vi "userTable.vi"() -> ()   [LabVIEW 2020, in "userLibrary.lvlib"]
uses:
  userLibrary.lvlib
  <vilib>/Utility/miscctls.llb/LVRowAndColumnTypeDef.ctl
  <vilib>/measure/mamon.llb/Trigger Detection for 1 Channel.vi
  <vilib>/addons/database/Connection.llb/DB Tools Open Connec (String).vi
  <vilib>/addons/database/NI_Database_API.lvlib
  databaseLibrary.lvlib
  maintenanceLibrary.lvlib
  <vilib>/measure/NI_MAPro.lvlib
panel:
  in  "close":bool
  out "status 5":bool
  out "status 4":bool
  out "status 3":bool
  out "status 2":bool
  out "status 1":bool
  out "Log Max row":i32
  in  "OK":bool
  in  "Change Pass":bool
  out "data":string[][](array[string])
  in  "Delete":bool
  in  "Update":bool
  in  "New":bool
  out "User Table":string[][](table) caption="Thickness Table"
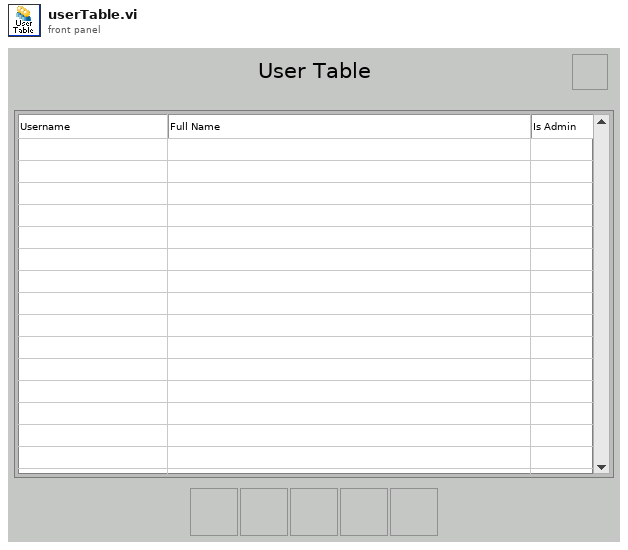
[diagram p1: front panel]
types:
  T1 = typedef "LVRowAndColumnTypeDef.ctl" = cluster{"Row":i32, "Column":i32}
  T2 = typedef "NI_Database_API.lvlib/Conn ObjectReference.ctl" = refnum<k1>
  T3 = cluster{"date/time string":string, "date/time string":string, "date/time string":string, string}
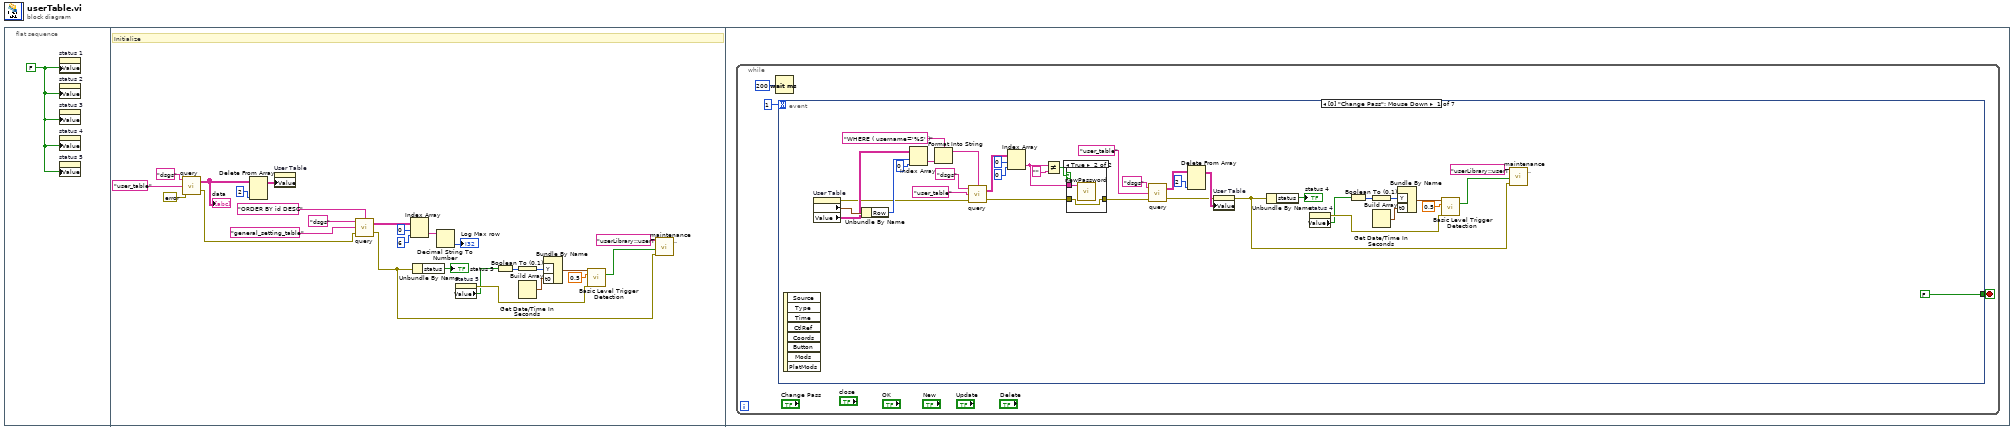
[diagram p0: block diagram]
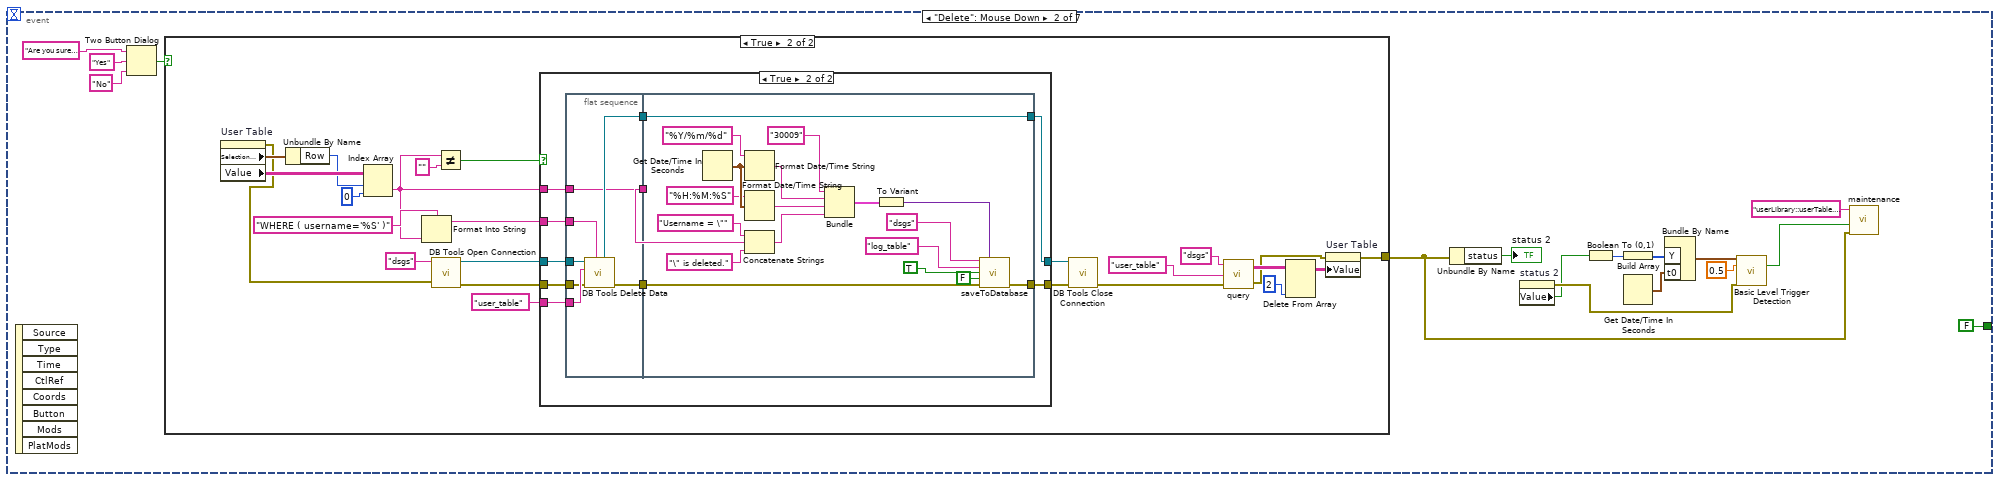
[diagram p3: hidden frame]
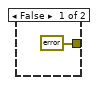
[diagram p4: hidden frame]
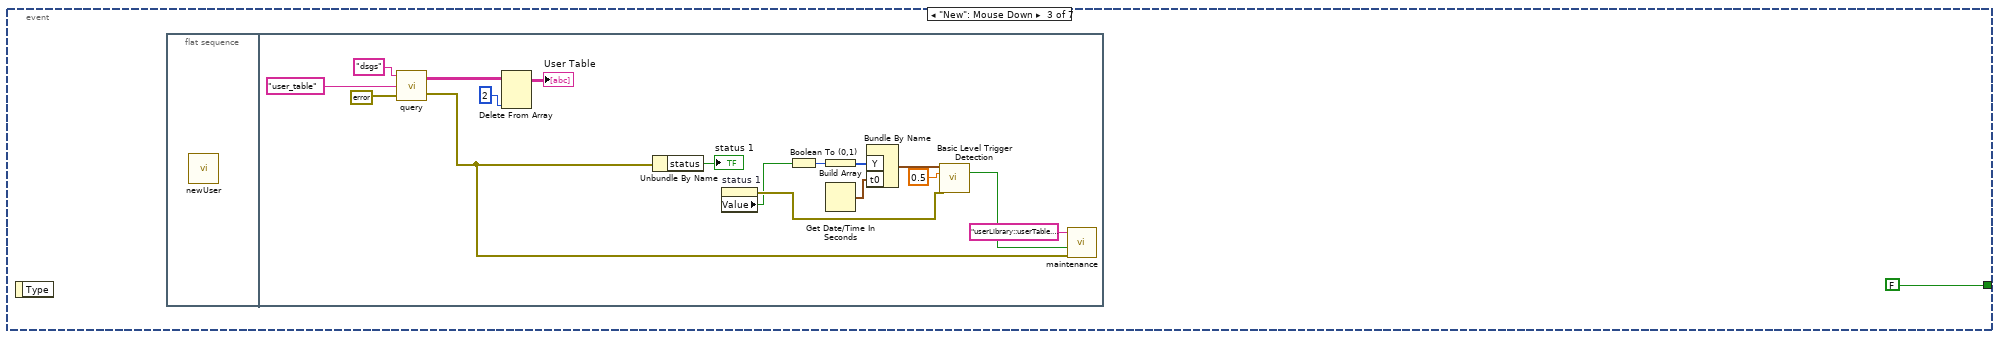
[diagram p6: hidden frame]
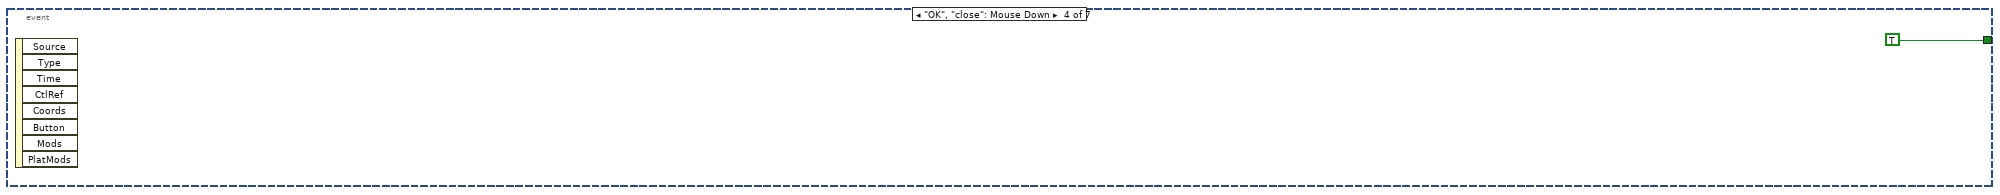
[diagram p7: hidden frame]
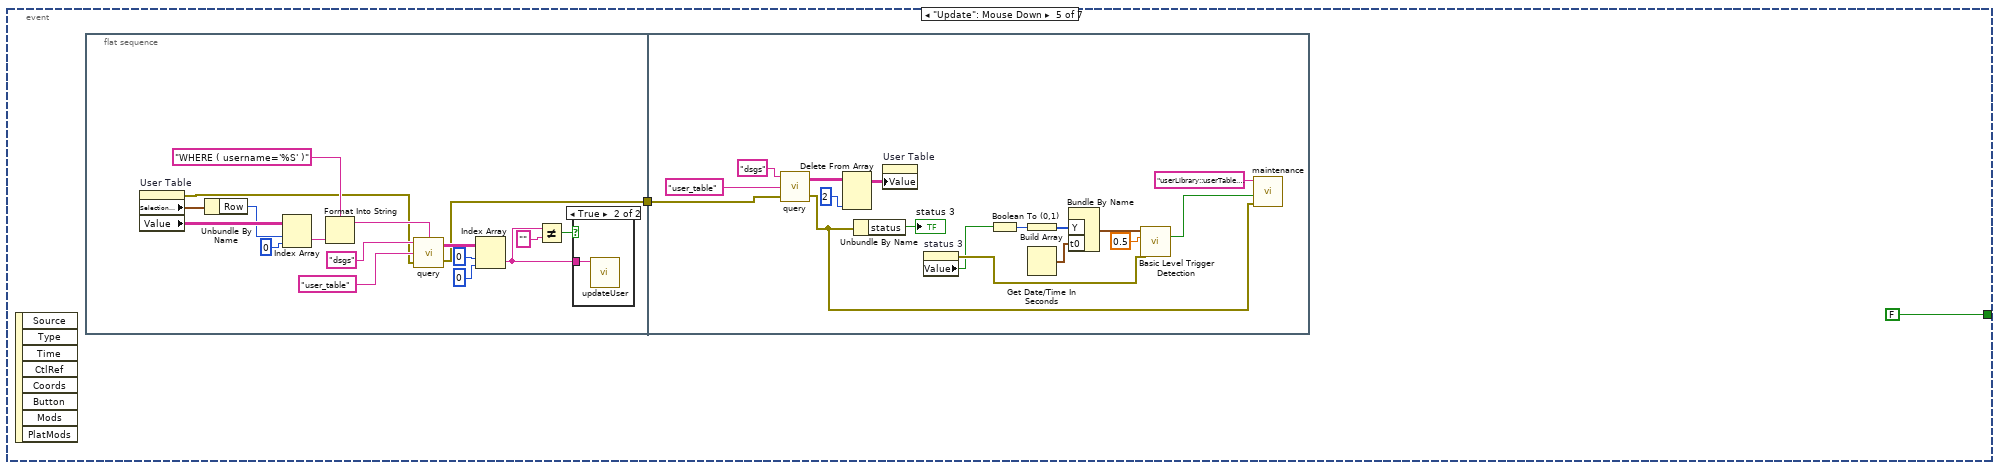
[diagram p8: hidden frame]
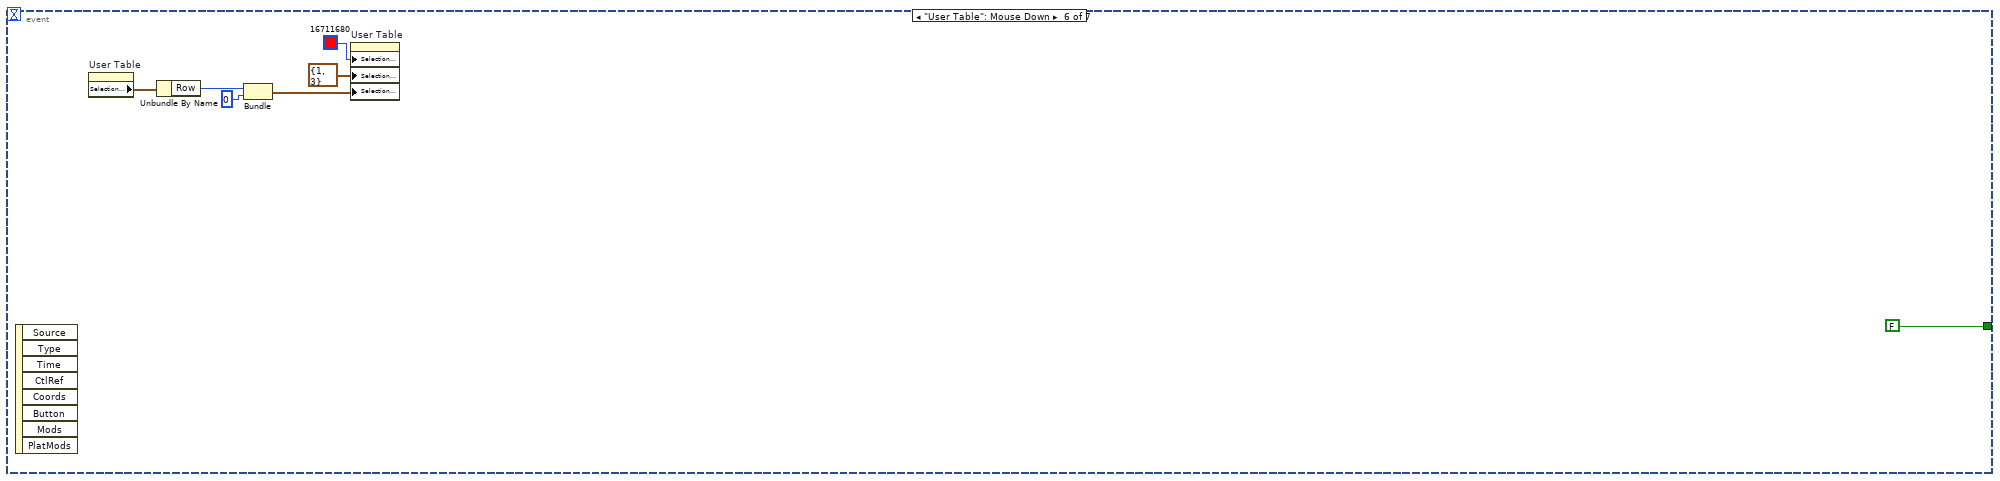
[diagram p10: hidden frame]
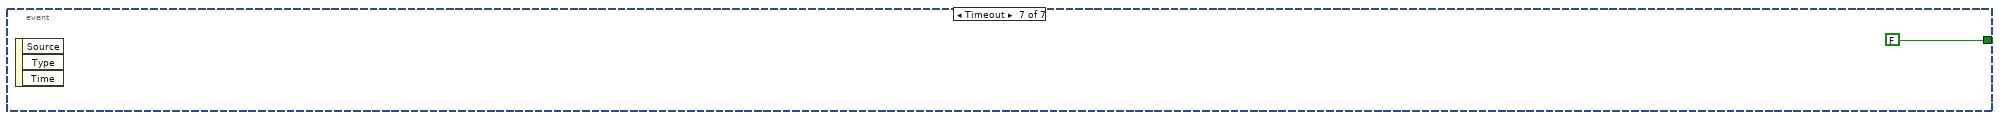
[diagram p11: hidden frame]
diagram:
  n1 = flat-sequence {
    frame #0 {
      w1 = FALSE ("status 1")
      n2 = property on="status 1" class="Bool (strict)"("Value"=w1) -> ()  [unwired: 2 in, 2 out]
      n3 = property on="status 2" class="Bool (strict)"("Value"=w1) -> ()  [unwired: 2 in, 2 out]
      n4 = property on="status 3" class="Bool (strict)"("Value"=w1) -> ()  [unwired: 2 in, 2 out]
      n5 = property on="status 4" class="Bool (strict)"("Value"=w1) -> ()  [unwired: 2 in, 2 out]
      n6 = property on="status 5" class="Bool (strict)"("Value"=w1) -> ()  [unwired: 2 in, 2 out]
    }
    frame #1 {
      # "Initialize"
      n7 = call "query.vi"("errorIn"=errorcluster {"status"=FALSE, "code"=0, "source"=""} ("Error in"), "Table Name"="user_table", "Connection Name"="dsgs") -> ("errorOut"=w14:errorcluster, "data"=w25:string[][])  [unwired: 1 in]
      "data" <- w25
      n8 = Delete From Array(array=w25, index (col)=2 ("disabled index (col)")) -> (array with subset deleted=w24:string[][])  [unwired: 2 in, 1 out]
      n9 = property on="User Table" class="Tbl (strict)"("Value"=w24) -> ()  [unwired: 2 in, 2 out]
      n10 = call "query.vi"("Condition"="ORDER BY id DESC", "errorIn"=w14, "Table Name"="general_setting_table", "Connection Name"="dsgs") -> ("errorOut"=w2:errorcluster, "data"=w22:string[][])
      n11 = Index Array(array=w22, index (row)=0, index (col)=6 ("disabled index (col)")) -> (element=w15:string)
      n12 = Unbundle By Name(w2) -> ("status"=→"status 5":bool)
      n13 = Decimal String To Number(string=w15) -> (number=→"Log Max row":i32)  [unwired: 2 in, 1 out]
      n14 = property on="status 5" class="Bool (strict)"() -> (error out=w10:errorcluster, "Value"=w9:bool)  [unwired: 2 in, 1 out]
      n15 = Boolean To (0,1)(Boolean=w9) -> (0, 1=w5:i16)
      n16 = Build Array(w5) -> (w7:i16[])
      n17 = Get Date/Time In Seconds() -> (seconds since 1Jan1904=w6:timestamp)
      n18 = Bundle By Name("Y"=w7, "t0"=w6) -> (w8:waveform(i16))  [unwired: 1 in]
      n19 = call-poly <vilib>:"Basic Level Trigger Detection.vi"("signal in"=w8, "level"=0.5, "error in (no error)"=w10) -> ("trigger detected?"=w11:bool)  [unwired: 10 in, 2 out]
      n20 = call "maintenance.vi"("errorIn"=w2, "status"=w11, "errorLocation"="userLibrary::userTable.vi::Initialize") -> ()  [unwired: 8 in, 1 out]
    }
    frame #2 {
      n21 = while {
        stop <- w28 stop-if-true
        n22 = Wait (ms)(milliseconds to wait=u32 200) -> ()  [unwired: 1 out]
        n23 = event shown="[0] \"Change Pass\": Mouse Down" {
          selector: _ -> [_ _ _ _ _ _ _]
          dyn-events: _ -> [_ _ _ _ _ _ _]
          timeout: 1 -> [_ _ _ _ _ _ _]
          tunnel: [FALSE FALSE FALSE TRUE FALSE FALSE FALSE] -> w28
          event "Change Pass": Mouse Down {
            n24 = event-data() -> ()  [unwired: 1 in, 8 out]
            n25 = property on="User Table" class="Tbl (strict)"() -> (error out=w43:errorcluster, "Selection Start"=w65:T1, "Value"=w64:string[][])  [unwired: 2 in, 1 out]
            n26 = Unbundle By Name(w65) -> ("Row"=w63:i32)
            n27 = Index Array(array=w64, index (row)=w63, index (col)=0 ("disabled index (col)")) -> (element=w66:string)
            n28 = Format Into String(format string="WHERE ( username='%S' )" ("condition"), w66) -> (resulting string=w60:string)  [unwired: 2 in, 1 out]
            n29 = call "query.vi"("Condition"=w60, "errorIn"=w43, "Table Name"="user_table", "Connection Name"="dsgs") -> ("errorOut"=w61:errorcluster, "data"=w59:string[][])
            n30 = Index Array(array=w59, index (row)=0, index (col)=0 ("disabled index (col)")) -> (element=w58:string)
            n31 = Not Equal?(x=w58, y="") -> (x != y?=w57:bool)
            n32 = case shown="True" w57 {
              tunnel: [w67 w68] -> w62
              tunnel: w61 -> [w67 w68]
              tunnel: w58 -> [_ w69]
              frame False {
              }
              frame True {
                n33 = call "newPassword.vi"("Username"=w69) -> ()  [unwired: 11 in]
              }
            }
            n34 = call "query.vi"("errorIn"=w62, "Table Name"="user_table", "Connection Name"="dsgs") -> ("errorOut"=w42:errorcluster, "data"=w56:string[][])  [unwired: 1 in]
            n35 = Delete From Array(array=w56, index (col)=2 ("disabled index (col)")) -> (array with subset deleted=w55:string[][])  [unwired: 2 in, 1 out]
            n36 = property on="User Table" class="Tbl (strict)"(error in=w42, "Value"=w55) -> (error out=w31:errorcluster)  [unwired: 1 in, 1 out]
            n37 = Unbundle By Name(w31) -> ("status"=→"status 4":bool)
            n38 = property on="status 4" class="Bool (strict)"() -> (error out=w39:errorcluster, "Value"=w38:bool)  [unwired: 2 in, 1 out]
            n39 = Boolean To (0,1)(Boolean=w38) -> (0, 1=w34:i16)
            n40 = Build Array(w34) -> (w36:i16[])
            n41 = Get Date/Time In Seconds() -> (seconds since 1Jan1904=w35:timestamp)
            n42 = Bundle By Name("Y"=w36, "t0"=w35) -> (w37:waveform(i16))  [unwired: 1 in]
            n43 = call-poly <vilib>:"Basic Level Trigger Detection.vi"("signal in"=w37, "level"=0.5, "error in (no error)"=w39) -> ("trigger detected?"=w40:bool)  [unwired: 10 in, 2 out]
            n44 = call "maintenance.vi"("errorIn"=w31, "status"=w40, "errorLocation"="userLibrary::userTable.vi::Change Pass case") -> ()  [unwired: 8 in, 1 out]
          }
          event "Delete": Mouse Down {
            n45 = event-data() -> ()  [unwired: 1 in, 8 out]
            n46 = Two Button Dialog(message="Are you sure to delete this user?", 1:"No" ("F button name (\"Cancel\")"), 2:"Yes" ("T button name (\"OK\")")) -> (T button?=w85:bool)
            n47 = case shown="True" w85 {
              tunnel: [errorcluster {"status"=FALSE, "code"=0, "source"=""} ("error out") w87] -> w70
              frame False {
              }
              frame True {
                n48 = property on="User Table" class="Tbl (strict)"() -> (error out=w89:errorcluster, "Selection Start"=w110:T1, "Value"=w105:string[][])  [unwired: 2 in, 1 out]
                n49 = Unbundle By Name(w110) -> ("Row"=w104:i32)
                n50 = Index Array(array=w105, index (row)=w104, index (col)=0 ("disabled index (col)")) -> (element=w90:string)
                n51 = Format Into String(format string="WHERE ( username='%S' )" ("condition"), w90) -> (resulting string=w97:string)  [unwired: 2 in, 1 out]
                n52 = call-poly <vilib>:"DB Tools Open Connection.vi"("error in (no error)"=w89, "connection information"="dsgs") -> ("error out"=w106:errorcluster, "connection reference"=w108:T2)  [unwired: 6 in]
                n53 = Not Equal?(x=w90, y="") -> (x != y?=w95:bool)
                n54 = case shown="True" w95 {
                  tunnel: w108 -> [w112 w122]
                  tunnel: "user_table" ("table") -> [_ w121]
                  tunnel: w106 -> [w111 w120]
                  tunnel: [w112 w119] -> w102
                  tunnel: [w111 w118] -> w101
                  tunnel: w97 -> [_ w117]
                  tunnel: w90 -> [_ w114]
                  frame False {
                  }
                  frame True {
                    n55 = flat-sequence {
                      tunnel: w122 -> [w129]
                      tunnel: w121 -> [w128]
                      tunnel: w120 -> [w127]
                      tunnel: w117 -> [w124]
                      tunnel: [w126] -> w116
                      tunnel: [w125] -> w115
                      tunnel: w114 -> [w123]
                      tunnel: [w123] -> w113
                      tunnel: [w136] -> w118
                      tunnel: [w148] -> w119
                      tunnel: w116 -> [w148]
                      tunnel: w115 -> [w131]
                      tunnel: w113 -> [w135]
                      frame #0 {
                        n56 = call <vilib>:"DB Tools Delete Data.vi"("condition"=w124, "error in (no error)"=w127, "table"=w128, "connection reference"=w129) -> ("error out"=w125:errorcluster, "connection reference out"=w126:T2)  [unwired: 6 in]
                      }
                      frame #1 {
                        n57 = Get Date/Time In Seconds() -> (seconds since 1Jan1904=w146:timestamp)
                        n58 = Format Date/Time String(time format string (%c)="%Y/%m/%d", seconds (now)=w146) -> (date/time string=w145:string)  [unwired: 1 in]
                        n59 = Format Date/Time String(time format string (%c)="%H:%M:%S", seconds (now)=w146) -> (date/time string=w144:string)  [unwired: 1 in]
                        n60 = Concatenate Strings("Username = \"" ("string"), w135, "\" is deleted." ("string")) -> (w147:string)
                        n61 = Bundle("date/time string"="30009", "date/time string"=w145, "date/time string"=w144, w147) -> (w143:T3)  [unwired: 1 in]
                        n62 = To Variant(anything=w143) -> (Variant=w142:variant)
                        n63 = call "saveToDatabase.vi"("Connection"="dsgs" ("table"), "Data"=w142, "Table"="log_table" ("table"), "Auto Increment ID?"=TRUE, "Delete row?"=FALSE, "Error in"=w131) -> ("Error out"=w136:errorcluster)  [unwired: 9 in]
                      }
                    }
                  }
                }
                n64 = call <vilib>:"DB Tools Close Connection.vi"("error in (no error)"=w101, "connection reference"=w102) -> ("error out"=w98:errorcluster)  [unwired: 5 in]
                n65 = call "query.vi"("errorIn"=w98, "Table Name"="user_table", "Connection Name"="dsgs") -> ("errorOut"=w88:errorcluster, "data"=w92:string[][])  [unwired: 1 in]
                n66 = Delete From Array(array=w92, index (col)=2 ("disabled index (col)")) -> (array with subset deleted=w91:string[][])  [unwired: 2 in, 1 out]
                n67 = property on="User Table" class="Tbl (strict)"(error in=w88, "Value"=w91) -> (error out=w87:errorcluster)  [unwired: 1 in, 1 out]
              }
            }
            n68 = Unbundle By Name(w70) -> ("status"=→"status 2":bool)
            n69 = property on="status 2" class="Bool (strict)"() -> (error out=w78:errorcluster, "Value"=w77:bool)  [unwired: 2 in, 1 out]
            n70 = Boolean To (0,1)(Boolean=w77) -> (0, 1=w73:i16)
            n71 = Build Array(w73) -> (w75:i16[])
            n72 = Get Date/Time In Seconds() -> (seconds since 1Jan1904=w74:timestamp)
            n73 = Bundle By Name("Y"=w75, "t0"=w74) -> (w76:waveform(i16))  [unwired: 1 in]
            n74 = call-poly <vilib>:"Basic Level Trigger Detection.vi"("signal in"=w76, "level"=0.5, "error in (no error)"=w78) -> ("trigger detected?"=w79:bool)  [unwired: 10 in, 2 out]
            n75 = call "maintenance.vi"("errorIn"=w70, "status"=w79, "errorLocation"="userLibrary::userTable.vi::Delete case") -> ()  [unwired: 8 in, 1 out]
          }
          event "New": Mouse Down {
            n76 = event-data() -> ()  [unwired: 1 in, 1 out]
            n77 = flat-sequence {
              frame #0 {
                n78 = call "newUser.vi"() -> ()  [unwired: 12 in]
              }
              frame #1 {
                n79 = call "query.vi"("errorIn"=errorcluster {"status"=FALSE, "code"=0, "source"=""} ("Error in"), "Table Name"="user_table", "Connection Name"="dsgs") -> ("errorOut"=w150:errorcluster, "data"=w164:string[][])  [unwired: 1 in]
                n80 = Delete From Array(array=w164, index (col)=2 ("disabled index (col)")) -> (array with subset deleted=→"User Table":string[][])  [unwired: 2 in, 1 out]
                n81 = Unbundle By Name(w150) -> ("status"=→"status 1":bool)
                n82 = property on="status 1" class="Bool (strict)"() -> (error out=w158:errorcluster, "Value"=w157:bool)  [unwired: 2 in, 1 out]
                n83 = Boolean To (0,1)(Boolean=w157) -> (0, 1=w153:i16)
                n84 = Build Array(w153) -> (w155:i16[])
                n85 = Get Date/Time In Seconds() -> (seconds since 1Jan1904=w154:timestamp)
                n86 = Bundle By Name("Y"=w155, "t0"=w154) -> (w156:waveform(i16))  [unwired: 1 in]
                n87 = call-poly <vilib>:"Basic Level Trigger Detection.vi"("signal in"=w156, "level"=0.5, "error in (no error)"=w158) -> ("trigger detected?"=w159:bool)  [unwired: 10 in, 2 out]
                n88 = call "maintenance.vi"("errorIn"=w150, "status"=w159, "errorLocation"="userLibrary::userTable.vi::New case") -> ()  [unwired: 8 in, 1 out]
              }
            }
          }
          event "OK", "close": Mouse Down {
            n89 = event-data() -> ()  [unwired: 1 in, 8 out]
          }
          event "Update": Mouse Down {
            n90 = event-data() -> ()  [unwired: 1 in, 8 out]
            n91 = flat-sequence {
              tunnel: [w171] -> w168
              tunnel: w168 -> [w199]
              frame #0 {
                n92 = property on="User Table" class="Tbl (strict)"() -> (error out=w170:errorcluster, "Selection Start"=w186:T1, "Value"=w185:string[][])  [unwired: 2 in, 1 out]
                n93 = Unbundle By Name(w186) -> ("Row"=w184:i32)
                n94 = Index Array(array=w185, index (row)=w184, index (col)=0 ("disabled index (col)")) -> (element=w183:string)
                n95 = Format Into String(format string="WHERE ( username='%S' )" ("condition"), w183) -> (resulting string=w178:string)  [unwired: 2 in, 1 out]
                n96 = call "query.vi"("Condition"=w178, "errorIn"=w170, "Table Name"="user_table", "Connection Name"="dsgs") -> ("errorOut"=w171:errorcluster, "data"=w177:string[][])
                n97 = Index Array(array=w177, index (row)=0, index (col)=0 ("disabled index (col)")) -> (element=w174:string)
                n98 = Not Equal?(x=w174, y="") -> (x != y?=w173:bool)
                n99 = case shown="True" w173 {
                  tunnel: w174 -> [_ w187]
                  frame False {
                  }
                  frame True {
                    n100 = call "updateUser.vi"("Username"=w187) -> ()  [unwired: 11 in]
                  }
                }
              }
              frame #1 {
                n101 = call "query.vi"("errorIn"=w199, "Table Name"="user_table", "Connection Name"="dsgs") -> ("errorOut"=w188:errorcluster, "data"=w203:string[][])  [unwired: 1 in]
                n102 = Delete From Array(array=w203, index (col)=2 ("disabled index (col)")) -> (array with subset deleted=w204:string[][])  [unwired: 2 in, 1 out]
                n103 = Unbundle By Name(w188) -> ("status"=→"status 3":bool)
                n104 = property on="User Table" class="Tbl (strict)"("Value"=w204) -> ()  [unwired: 2 in, 2 out]
                n105 = property on="status 3" class="Bool (strict)"() -> (error out=w196:errorcluster, "Value"=w195:bool)  [unwired: 2 in, 1 out]
                n106 = Boolean To (0,1)(Boolean=w195) -> (0, 1=w191:i16)
                n107 = Build Array(w191) -> (w193:i16[])
                n108 = Get Date/Time In Seconds() -> (seconds since 1Jan1904=w192:timestamp)
                n109 = Bundle By Name("Y"=w193, "t0"=w192) -> (w194:waveform(i16))  [unwired: 1 in]
                n110 = call-poly <vilib>:"Basic Level Trigger Detection.vi"("signal in"=w194, "level"=0.5, "error in (no error)"=w196) -> ("trigger detected?"=w197:bool)  [unwired: 10 in, 2 out]
                n111 = call "maintenance.vi"("errorIn"=w188, "status"=w197, "errorLocation"="userLibrary::userTable.vi::Update case") -> ()  [unwired: 8 in, 1 out]
              }
            }
          }
          event "User Table": Mouse Down {
            n112 = event-data() -> ()  [unwired: 1 in, 8 out]
            n113 = property on="User Table" class="Tbl (strict)"() -> ("Selection Start"=w208:T1)  [unwired: 2 in, 2 out]
            n114 = Unbundle By Name(w208) -> ("Row"=w209:i32)
            n115 = Bundle("Row"=w209, "Row"=0) -> (w211:cluster{"Row":i32, "Row":i32})  [unwired: 1 in]
            n116 = property on="User Table" class="Tbl (strict)"("Selection Color"=u32 16711680, "Selection Size"=T1 {"Row"=1, "Column"=3}, "Selection Start"=w211) -> ()  [unwired: 2 in, 2 out]
          }
          event Timeout {
            n117 = event-data() -> ()  [unwired: 1 in, 3 out]
          }
        }
      }
    }
  }
